vi "Initialize Work.vi"(8 "error in (no error)":errorcluster, 9 "Update period":dbl, 10 "Reply to":refnum<class "Result Reply Msg.lvclass">, 11 "Measure Object in":refnum<class "Simple Sequencer.lvclass">) -> (0 "error out":errorcluster, 3 "Measure Object out":refnum<class "Simple Sequencer.lvclass">)   [LabVIEW 2018, in "Simple Sequencer.lvclass"]
uses:
  Simple Sequencer.lvclass
  Template Module Messages/Result Reply Msg/Result Reply Msg.lvclass
  NHMFL_Core/Libraries/Instruments/Sequence/Sequencer State Machine/Sequencer State.ctl
  Worker/Worker.lvclass
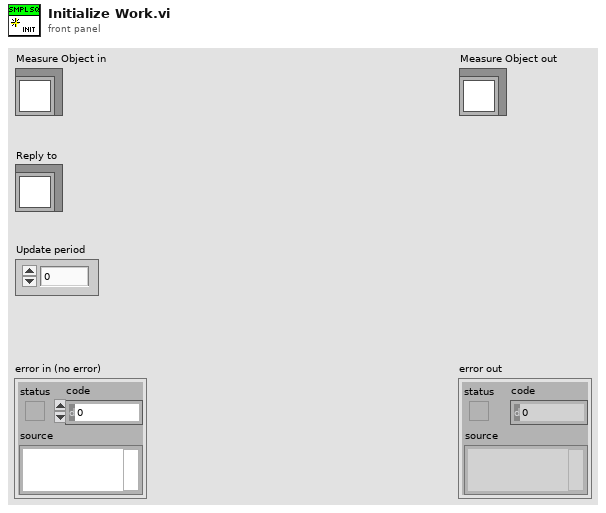
[diagram p1: front panel]
types:
  T1 = typedef "Sequencer State.ctl" = enum16{"Idle", "Starting", "Waiting for primary", "Waiting for secondary"}
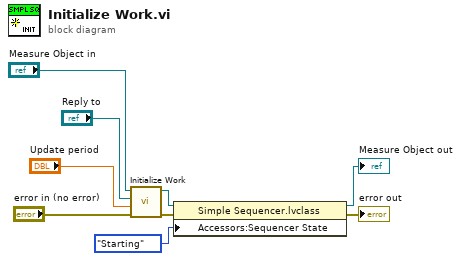
[diagram p0: block diagram]
diagram:
  n1 = call-parent "Initialize Work.vi"("error in (no error)"="error in (no error)", "Update period"="Update period", "Reply to"="Reply to", "Measure Object in"="Measure Object in") -> ("error out"=w2:errorcluster, "Measure Object out"=w4:refnum<class "Simple Sequencer.lvclass">)  [unwired: 6 in]
  n2 = property class="Simple Sequencer.lvclass"(reference=w4, error in=w2, "Accessors:Sequencer State"=Sequencer_State."Starting" ("Sequencer State")) -> (reference out=→"Measure Object out":refnum<class "Simple Sequencer.lvclass">, error out=→"error out":errorcluster)
